vi "aw_WRDCluster_8acel_baja_velocidad.vi"(4 "TimeStamp":dbl, 5 "p_tp":dbl, 6 "p_sp":dbl, 7 "Array TAGs":string[](array[string]), 8 "Energía":dbl[][](array[numeric]), 9 "Amplitudes":dbl[][](array[numeric]), 10 "Frecuencia Ruedas":dbl[][](array[numeric]), 11 "Max RMS Ruedas":dbl[][](array[numeric])) -> (1 "JSON cluster":T1)   [LabVIEW 2015]
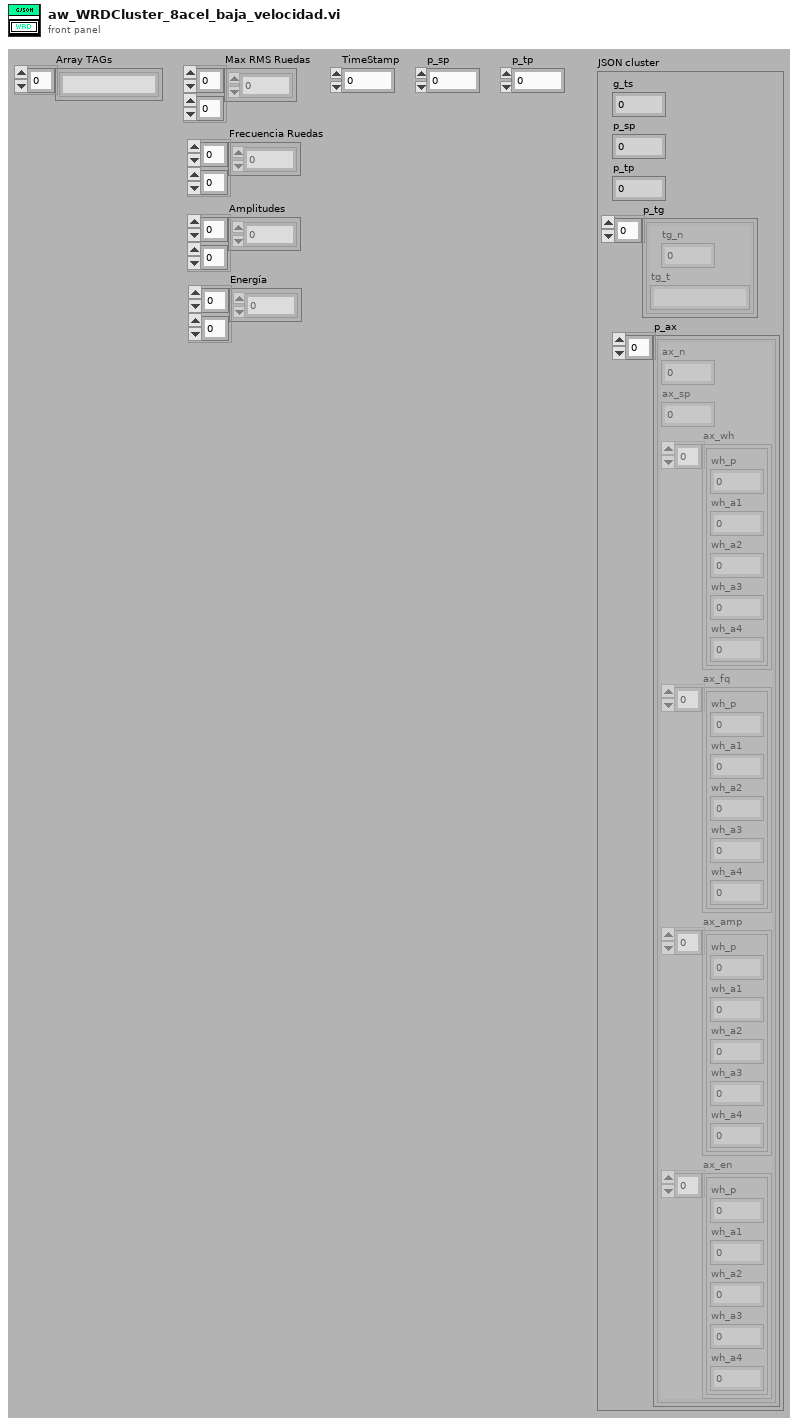
[diagram p1: front panel]
types:
  T1 = cluster{"g_ts":dbl, "p_sp":dbl, "p_tp":dbl, "p_tg":cluster{"tg_n":dbl, "tg_t":string}[], "p_ax":cluster{"ax_n":dbl, "ax_sp":dbl, "ax_wh":cluster{"wh_p":dbl, "wh_a1":dbl, "wh_a2":dbl, "wh_a3":dbl, "wh_a4":dbl}[], "ax_fq":cluster{"wh_p":dbl, "wh_a1":dbl, "wh_a2":dbl, "wh_a3":dbl, "wh_a4":dbl}[], "ax_amp":cluster{"wh_p":dbl, "wh_a1":dbl, "wh_a2":dbl, "wh_a3":dbl, "wh_a4":dbl}[], "ax_en":cluster{"wh_p":dbl, "wh_a1":dbl, "wh_a2":dbl, "wh_a3":dbl, "wh_a4":dbl}[]}[]}
  T2 = cluster{"wh_p":dbl, "wh_a1":dbl, "wh_a2":dbl, "wh_a3":dbl, "wh_a4":dbl}
  T3 = cluster{"ax_n":dbl, "ax_sp":dbl, "ax_wh":cluster{"wh_p":dbl, "wh_a1":dbl, "wh_a2":dbl, "wh_a3":dbl, "wh_a4":dbl}[], "ax_fq":cluster{"wh_p":dbl, "wh_a1":dbl, "wh_a2":dbl, "wh_a3":dbl, "wh_a4":dbl}[], "ax_amp":cluster{"wh_p":dbl, "wh_a1":dbl, "wh_a2":dbl, "wh_a3":dbl, "wh_a4":dbl}[], "ax_en":cluster{"wh_p":dbl, "wh_a1":dbl, "wh_a2":dbl, "wh_a3":dbl, "wh_a4":dbl}[]}
  T4 = cluster{"wh_p":dbl, "wh_a1":dbl, "wh_a2":dbl, "wh_a3":dbl, "wh_a4":dbl}[]
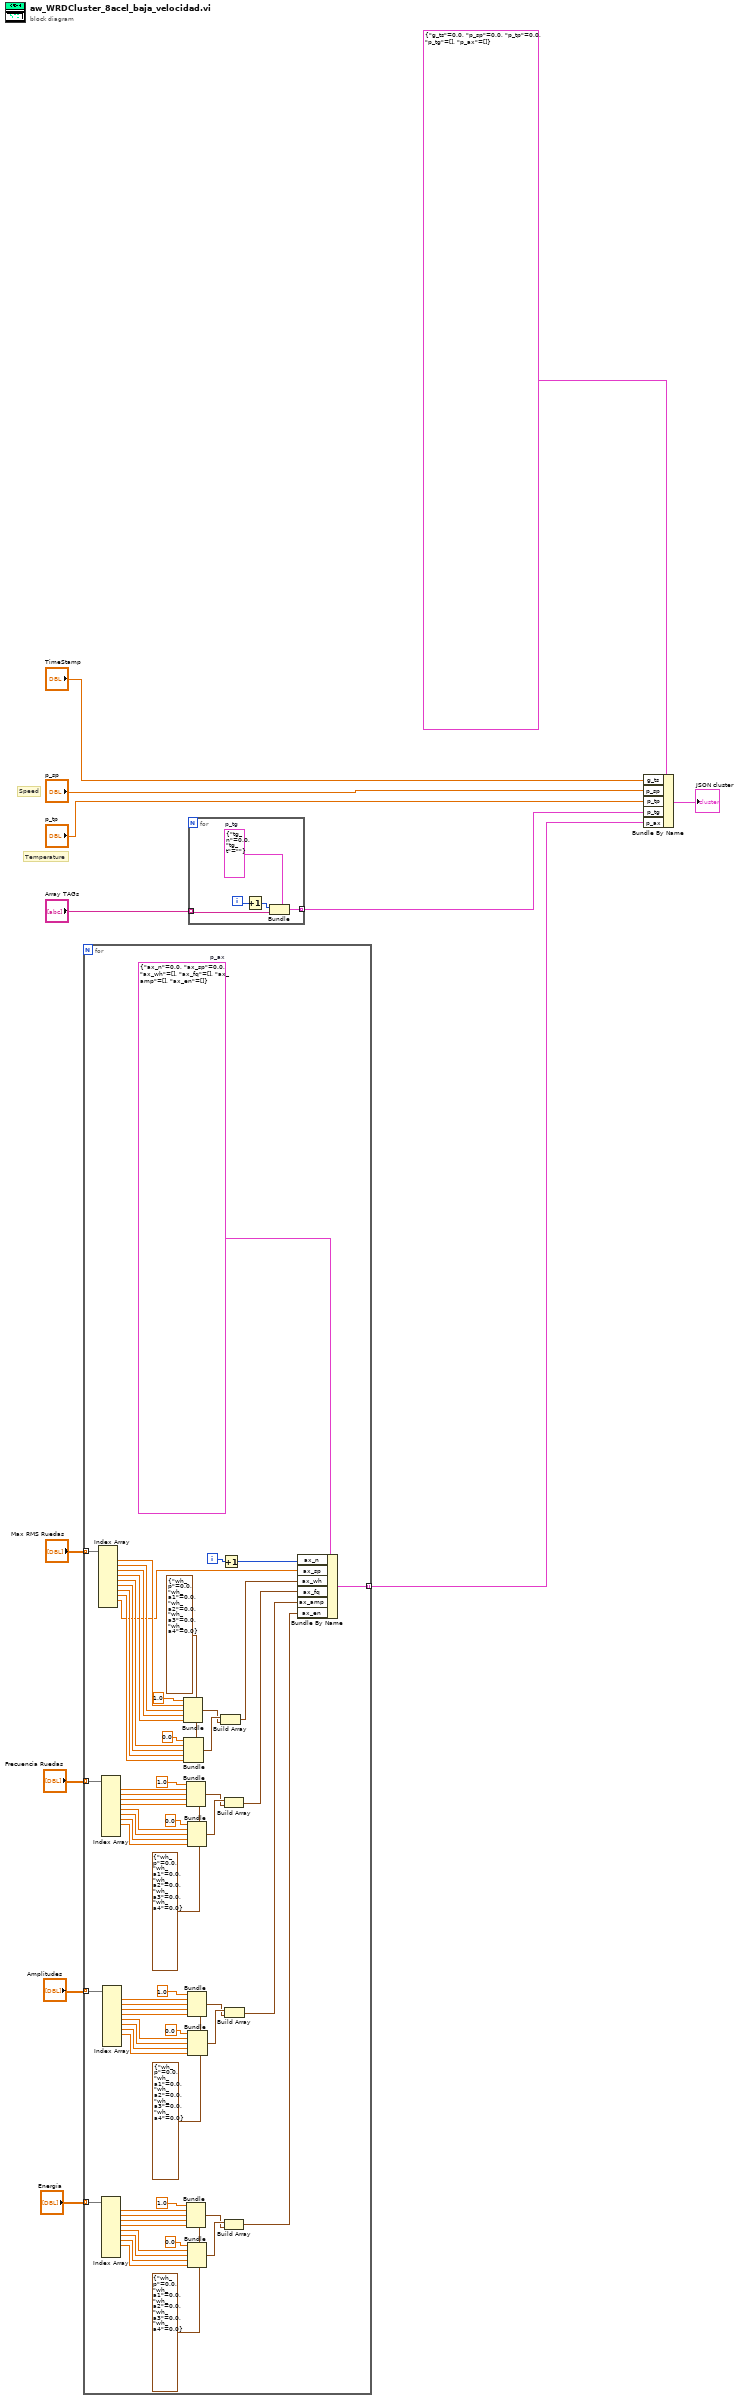
[diagram p0: block diagram]
diagram:
  # "Speed"
  # "Temperature"
  n1 = for {
    tunnel: "Max RMS Ruedas" -> [w77] mode=indexing
    tunnel: [w68] -> w7 mode=indexing
    tunnel: "Frecuencia Ruedas" -> [w45] mode=indexing
    tunnel: "Amplitudes" -> [w30] mode=indexing
    tunnel: "Energía" -> [w16] mode=indexing
    i -> [w75]
    w17 = T2 {"wh_p"=0.0, "wh_a1"=0.0, "wh_a2"=0.0, "wh_a3"=0.0, "wh_a4"=0.0} ("ax_wh")
    w31 = T2 {"wh_p"=0.0, "wh_a1"=0.0, "wh_a2"=0.0, "wh_a3"=0.0, "wh_a4"=0.0} ("ax_wh")
    w44 = T2 {"wh_p"=0.0, "wh_a1"=0.0, "wh_a2"=0.0, "wh_a3"=0.0, "wh_a4"=0.0} ("ax_wh")
    w67 = T2 {"wh_p"=0.0, "wh_a1"=0.0, "wh_a2"=0.0, "wh_a3"=0.0, "wh_a4"=0.0} ("ax_wh")
    w76 = T3 {"ax_n"=0.0, "ax_sp"=0.0, "ax_wh"=[], "ax_fq"=[], "ax_amp"=[], "ax_en"=[]}  # p_ax
    n2 = Index Array(array=w77) -> (element #1=w72:dbl, element #2=w70:dbl, element #3=w64:dbl, element #4=w63:dbl, element #5=w62:dbl, element #6=w61:dbl, element #7=w60:dbl, element #8=w59:dbl, element #9=w58:dbl)  [unwired: 10 in, 1 out]
    n3 = Index Array(array=w45) -> (element #1=w56:dbl, element #2=w54:dbl, element #3=w51:dbl, element #4=w50:dbl, element #5=w49:dbl, element #6=w48:dbl, element #7=w47:dbl, element #8=w46:dbl)  [unwired: 10 in, 2 out]
    n4 = Index Array(array=w16) -> (element #1=w28:dbl, element #2=w26:dbl, element #3=w23:dbl, element #4=w22:dbl, element #5=w21:dbl, element #6=w20:dbl, element #7=w19:dbl, element #8=w18:dbl)  [unwired: 10 in, 2 out]
    n5 = Index Array(array=w30) -> (element #1=w42:dbl, element #2=w40:dbl, element #3=w37:dbl, element #4=w36:dbl, element #5=w35:dbl, element #6=w34:dbl, element #7=w33:dbl, element #8=w32:dbl)  [unwired: 10 in, 2 out]
    n6 = Bundle(cluster=w67, "wh_p"=1.0, "wh_a1"=w72, "wh_a2"=w70, "wh_a3"=w64, "wh_a4"=w63) -> (w65:T2)
    n7 = Bundle(cluster=w67, "wh_p"=0.0, "wh_a1"=w62, "wh_a2"=w61, "wh_a3"=w60, "wh_a4"=w59) -> (w66:T2)
    n8 = Bundle(cluster=w44, "wh_p"=1.0, "wh_a1"=w56, "wh_a2"=w54, "wh_a3"=w51, "wh_a4"=w50) -> (w52:T2)
    n9 = Bundle(cluster=w17, "wh_p"=1.0, "wh_a1"=w28, "wh_a2"=w26, "wh_a3"=w23, "wh_a4"=w22) -> (w24:T2)
    n10 = Bundle(cluster=w44, "wh_p"=0.0, "wh_a1"=w49, "wh_a2"=w48, "wh_a3"=w47, "wh_a4"=w46) -> (w53:T2)
    n11 = Bundle(cluster=w31, "wh_p"=1.0, "wh_a1"=w42, "wh_a2"=w40, "wh_a3"=w37, "wh_a4"=w36) -> (w38:T2)
    n12 = Bundle(cluster=w17, "wh_p"=0.0, "wh_a1"=w21, "wh_a2"=w20, "wh_a3"=w19, "wh_a4"=w18) -> (w25:T2)
    n13 = Bundle(cluster=w31, "wh_p"=0.0, "wh_a1"=w35, "wh_a2"=w34, "wh_a3"=w33, "wh_a4"=w32) -> (w39:T2)
    n14 = Build Array(w66, w65) -> (w69:T4)
    n15 = Increment(x=w75) -> (x+1=w74:i32)
    n16 = Build Array(w53, w52) -> (w15:T4)
    n17 = Build Array(w25, w24) -> (w13:T4)
    n18 = Build Array(w39, w38) -> (w14:T4)
    n19 = Bundle By Name(cluster=w76, "ax_n"=w74, "ax_sp"=w58, "ax_wh"=w69, "ax_fq"=w15, "ax_amp"=w14, "ax_en"=w13) -> (w68:T3)
  }
  n20 = for {
    tunnel: "Array TAGs" -> [w79] mode=indexing
    tunnel: [w78] -> w12 mode=indexing
    i -> [w80]
    w82 = cluster{"tg_n":dbl, "tg_t":string} {"tg_n"=0.0, "tg_t"=""}  # p_tg
    n21 = Increment(x=w80) -> (x+1=w81:i32)
    n22 = Bundle(cluster=w82, "tg_n"=w81, "tg_t"=w79) -> (w78:cluster{"tg_n":dbl, "tg_t":string})
  }
  n23 = Bundle By Name(cluster=T1 {"g_ts"=0.0, "p_sp"=0.0, "p_tp"=0.0, "p_tg"=[], "p_ax"=[]}, "g_ts"="TimeStamp", "p_sp"="p_sp", "p_tp"="p_tp", "p_tg"=w12, "p_ax"=w7) -> (→"JSON cluster":T1)
